vi "travelDistanceWithCarpet.vi"(6 "Exclude Array":T1[](array[typedef]) {"Sizes"."Min" format="%#.1f"; "Sizes"."Max" format="%#.1f"}, 7 "moveCostWeighting":sgl[](array[numeric])=[1.0, 1.0, 1.0], 10 "pointB":sgl[](array[numeric]), 11 "pointA":sgl[](array[numeric])) -> (1 "distance":dbl, 2 "moveType":string)   [LabVIEW 2021]
uses:
  Route mapping/Exclude_cluster.ctl
  Route mapping/Box_size.ctl
  Route mapping/Exclusion_type.ctl
  <vilib>/Analysis/baseanly.llb/Real Dot Product.vi
  <vilib>/Analysis/NI_AALBase.lvlib
panel:
  # "Computes path length between points, taking account of \"Vertical Move Only\" carpet depth"
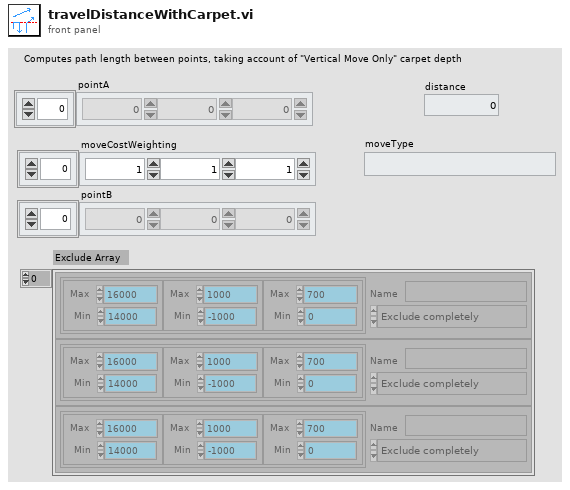
[diagram p1: front panel]
types:
  T1 = typedef "Exclude_cluster.ctl" = cluster{"Sizes":T2, "Name":string, "Exclude Type":T3}
  T2 = typedef "Box_size.ctl" = cluster{"Max":sgl, "Min":sgl}[]
  T3 = typedef "Exclusion_type.ctl" = enum16{"Exclude completely", "Allow only vertical moves"}
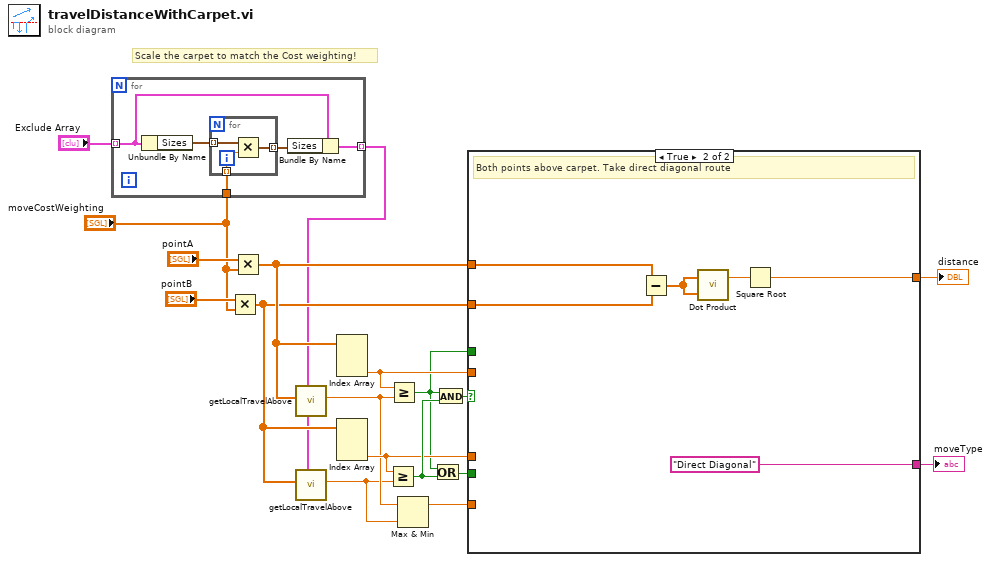
[diagram p0: block diagram]
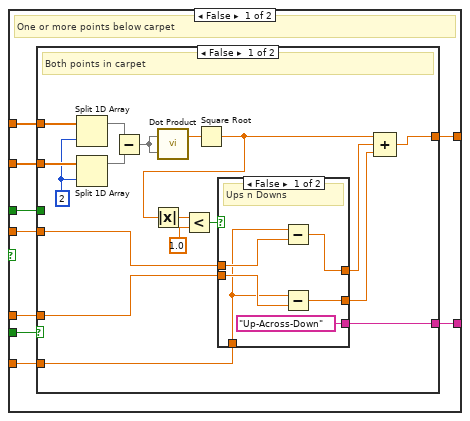
[diagram p2: hidden frame]
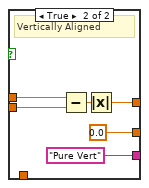
[diagram p3: hidden frame]
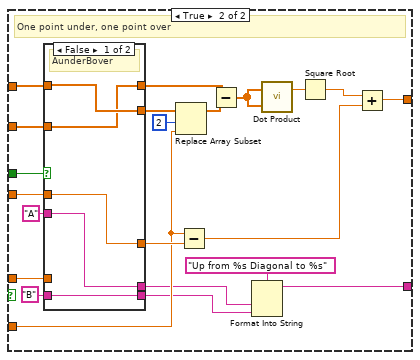
[diagram p4: hidden frame]
diagram:
  # "Scale the carpet to match the Cost weighting!"
  n1 = for {
    tunnel: "Exclude Array" -> [w21] mode=indexing
    tunnel: "moveCostWeighting" -> [w22]
    tunnel: [w19] -> w1 mode=indexing
    n2 = Unbundle By Name(w21) -> ("Sizes"=w23:T2)
    n3 = for {
      tunnel: w23 -> [w25] mode=indexing
      tunnel: w22 -> [w26] mode=indexing
      tunnel: [w24] -> w20 mode=indexing
      n4 = Multiply(x=w25, y=w26) -> (x*y=w24:cluster{"Max":sgl, "Min":sgl})
    }
    n5 = Bundle By Name(cluster=w21, "Sizes"=w20) -> (w19:T1)
  }
  n6 = Multiply(x="pointB", y="moveCostWeighting") -> (x*y=w4:sgl[])
  n7 = Multiply(x="pointA", y="moveCostWeighting") -> (x*y=w5:sgl[])
  n8 = call "getLocalTravelAbove.vi"("Exclude Array"=w1, "pointA"=w5) -> ("travelAboveHeight"=w8:sgl)  [unwired: 9 in]
  n9 = call "getLocalTravelAbove.vi"("Exclude Array"=w1, "pointA"=w4) -> ("travelAboveHeight"=w7:sgl)  [unwired: 9 in]
  n10 = Index Array(array=w5) -> (element #3=w14:sgl)  [unwired: 3 in, 2 out]
  n11 = Index Array(array=w4) -> (element #3=w13:sgl)  [unwired: 3 in, 2 out]
  n12 = Greater Or Equal?(x=w13, y=w7) -> (x >= y?=w16:bool)
  n13 = Greater Or Equal?(x=w14, y=w8) -> (x >= y?=w12:bool)
  n14 = Max & Min(x=w8, y=w7) -> (max(x,y)=w6:sgl)  [unwired: 1 out]
  n15 = Or(x=w12, y=w16) -> (x .or. y?=w15:bool)
  n16 = And(x=w12, y=w16) -> (x .and. y?=w17:bool)
  n17 = case shown="True" w17 {
    tunnel: [w29 w101] -> w18
    tunnel: w4 -> [w30 w100]
    tunnel: w5 -> [w31 w99]
    tunnel: w15 -> [w35 _]
    tunnel: w14 -> [w34 _]
    tunnel: w6 -> [w33 _]
    tunnel: w13 -> [w32 _]
    tunnel: w12 -> [w28 _]
    tunnel: [w27 "Direct Diagonal" ("moveType")] -> w11
    frame False {
      # "One or more points below carpet"
      n18 = case shown="False" w35 {
        tunnel: w34 -> [w53 w81]
        tunnel: w33 -> [w51 w80]
        tunnel: w32 -> [w52 w79]
        tunnel: w31 -> [w49 w86]
        tunnel: w30 -> [w48 w84]
        tunnel: [w41 w73] -> w29
        tunnel: w28 -> [_ w87]
        tunnel: [w36 w70] -> w27
        frame False {
          w47 = 2 ("index")
          # "Both points in carpet"
          n19 = Split 1D Array(array=w49, index=w47) -> (first subarray=w46:sgl[])  [unwired: 1 out]
          n20 = Split 1D Array(array=w48, index=w47) -> (first subarray=w45:sgl[])  [unwired: 1 out]
          n21 = Subtract(x=w46, y=w45) -> (x-y=w44:sgl[])
          n22 = call-poly <vilib>:"Dot Product.vi"("Y Vector"=w44, "X Vector"=w44) -> ("X * Y"=w50:dbl)  [unwired: 1 out]
          n23 = Square Root(x=w50) -> (sqrt(x)=w40:dbl)
          n24 = Absolute Value(x=w40) -> (abs(x)=w38:dbl)
          n25 = Less?(x=w38, y=1.0) -> (x < y?=w39:bool)
          n26 = case shown="False" w39 {
            tunnel: w53 -> [w59 w65]
            tunnel: w52 -> [w58 w64]
            tunnel: w51 -> [w57 _]
            tunnel: [w56 w62] -> w43
            tunnel: [w55 sgl 0.0] -> w42
            tunnel: ["Up-Across-Down" "Pure Vert"] -> w36
            frame False {
              # "Ups n Downs"
              n27 = Subtract(x=w57, y=w59) -> (x-y=w56:sgl)
              n28 = Subtract(x=w57, y=w58) -> (x-y=w55:sgl)
            }
            frame True {
              # "Vertically Aligned"
              n29 = Subtract(x=w65, y=w64) -> (x-y=w63:sgl)
              n30 = Absolute Value(x=w63) -> (abs(x)=w62:sgl)
            }
          }
          n31 = Compound Arithmetic op=ADD(w40, w43, w42) -> (w41:dbl)
        }
        frame True {
          # "One point under, one point over"
          n32 = case shown="False" w87 {
            tunnel: w86 -> [w92 w95]
            tunnel: w84 -> [w90 w97]
            tunnel: [w92 w97] -> w83
            tunnel: [w91 w96] -> w82
            tunnel: w81 -> [w91 _]
            tunnel: w79 -> [_ w96]
            tunnel: [w90 w95] -> w76
            tunnel: [w89 w94] -> w69
            tunnel: "A" -> [w89 w93]
            tunnel: "B" -> [w88 w94]
            tunnel: [w88 w93] -> w66
            frame False {
              # "AunderBover"
            }
            frame True {
              # "AoverBunder"
            }
          }
          n33 = Replace Array Subset(array=w83, new element=w80, index=2) -> (w75:sgl[])
          n34 = Subtract(x=w80, y=w82) -> (x-y=w72:sgl)
          n35 = Subtract(x=w76, y=w75) -> (x-y=w77:sgl[])
          n36 = Format Into String(format string="Up from %s Diagonal to %s", w69, w66) -> (resulting string=w70:string)  [unwired: 2 in, 1 out]
          n37 = call-poly <vilib>:"Dot Product.vi"("Y Vector"=w77, "X Vector"=w77) -> ("X * Y"=w78:dbl)  [unwired: 1 out]
          n38 = Square Root(x=w78) -> (sqrt(x)=w74:dbl)
          n39 = Add(x=w74, y=w72) -> (x+y=w73:dbl)
        }
      }
    }
    frame True {
      # "Both points above carpet. Take direct diagonal route"
      n40 = Subtract(x=w99, y=w100) -> (x-y=w102:sgl[])
      n41 = call-poly <vilib>:"Dot Product.vi"("Y Vector"=w102, "X Vector"=w102) -> ("X * Y"=w103:dbl)  [unwired: 1 out]
      n42 = Square Root(x=w103) -> (sqrt(x)=w101:dbl)
    }
  }
  "distance" <- w18
  "moveType" <- w11
